vi "NodMcu interlink labview.vi"() -> ()   [LabVIEW 2015]
panel:
  out "ultrasonic range":dbl(graph)
  out "data out":string
  out "Voltage(0-3.3v)":dbl(graph)
  in  "stop":bool
  out "Voltage":string
  in  "address":string
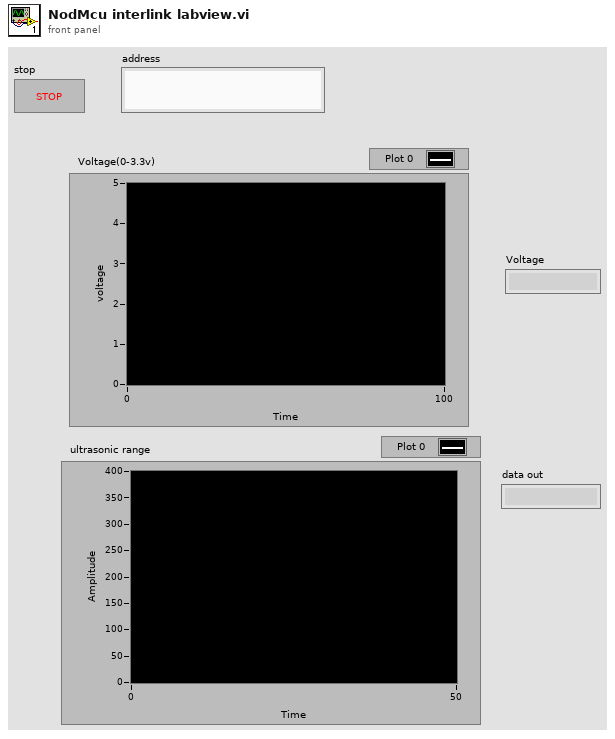
[diagram p1: front panel]
types:
  T1 = enum16{"Standard", "Buffered", "CRLF", "Immediate"}
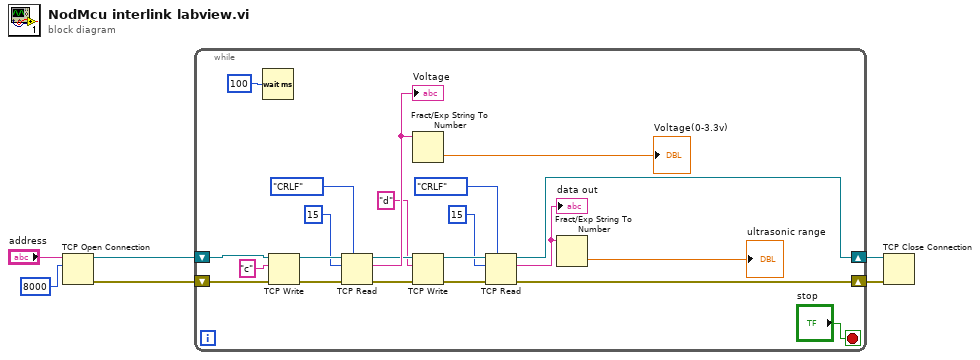
[diagram p0: block diagram]
diagram:
  n1 = TCP Open Connection(address="address", remote port or service name=u16 8000) -> (connection ID=w4:refnum<k5>, error out=w3:errorcluster)  [unwired: 3 in]
  n2 = while {
    shift-right: [w15] -> w2
    shift-left: w4 -> [w28]
    shift-right: [w12] -> w1
    shift-left: w3 -> [w27]
    stop <- "stop" stop-if-true
    n3 = Wait (ms)(milliseconds to wait=u32 100) -> ()  [unwired: 1 out]
    n4 = TCP Write(connection ID=w28, data in="c", error in (no error)=w27) -> (connection ID out=w26:refnum<k5>, error out=w25:errorcluster)  [unwired: 1 in, 1 out]
    n5 = TCP Read(connection ID=w26, bytes to read=15, error in (no error)=w25, 7:T1."CRLF" ("mode (standard)")) -> (connection ID out=w17:refnum<k5>, data out=w21:string, error out=w14:errorcluster)  [unwired: 1 in]
    "Voltage" <- w21
    n6 = Fract/Exp String To Number(string=w21) -> (number=→"Voltage(0-3.3v)":dbl)  [unwired: 3 in, 1 out]
    n7 = TCP Write(connection ID=w17, data in="d", error in (no error)=w14) -> (connection ID out=w16:refnum<k5>, error out=w13:errorcluster)  [unwired: 1 in, 1 out]
    n8 = TCP Read(connection ID=w16, bytes to read=15, error in (no error)=w13, 7:T1."CRLF" ("mode (standard)")) -> (connection ID out=w15:refnum<k5>, data out=w9:string, error out=w12:errorcluster)  [unwired: 1 in]
    "data out" <- w9
    n9 = Fract/Exp String To Number(string=w9) -> (number=→"ultrasonic range":dbl)  [unwired: 3 in, 1 out]
  }
  n10 = TCP Close Connection(connection ID=w2, error in (no error)=w1) -> ()  [unwired: 1 in, 2 out]
